vi "AprilTagPoseEstimator_Globals.vi"() -> ()   [LabVIEW 2019, in "Trajectory_Library.lvlib"]
doc: "Pose estimator configuration for AprilTag tags.\n\nContains:\n\n -- tagSize -- double -- tag size, in meters\n -- fx -- double -- camera horizontal focal length, in pixels\n -- fy -- double -- camera vertical focal length, in pixels\n -- cx -- double -- camera horizontal focal center, in pixels\n -- cy -- double -- camera vertical focal center, in pixels"
uses:
  Trajectory_Library.lvlib
panel:
  in  "Cy_pix":dbl
  in  "Cx_pix":dbl
  in  "Fy_pix":dbl
  in  "Fx_pix":dbl
  in  "TagSize_m":dbl
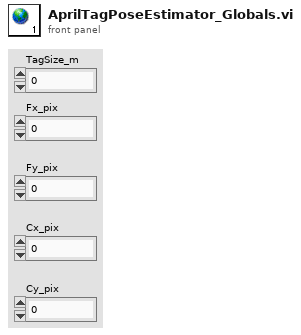
[diagram p1: front panel]
diagram:
